vi "Call.vi"(7 "Actor in":refnum<class "Actor.lvclass">, 8 "Error in":errorcluster, 9 "Error":errorcluster, 10 "Actor":refnum<class "Actor.lvclass">) -> (0 "Error out":errorcluster, 5 "Actor out":refnum<class "Actor.lvclass">)   [LabVIEW 2025, in "jettl.lvlib" / "Stopped jettl Msg.lvlib"]
uses:
  Stopped jettl Msg.lvlib
  Stopped Msg/Stopped Msg/Stopped Msg.lvclass
  C:/git/jettl/src/jettl/jettl/Stopped jettl Msg/--Stopped Msg/Stopped Msg.lvclass
  C:/git/jettl/src/jettl/jettl/Msg/Msg.lvclass
  jettl.lvlib
  Stopped Msg Output/Stopped Msg Output/Stopped Msg Output.lvclass
  Actor/Actor.lvclass
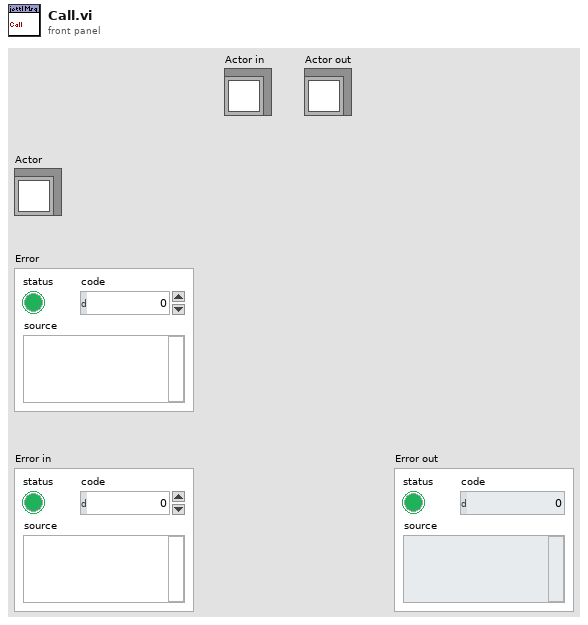
[diagram p1: front panel]
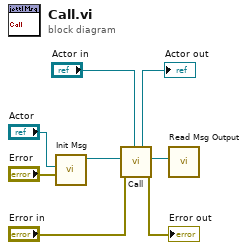
[diagram p0: block diagram]
diagram:
  n1 = call "Init Msg.vi"("Error"="Error", "Actor"="Actor") -> ("Stopped Msg out"=w6:refnum<class "Stopped Msg.lvclass">)  [unwired: 9 in]
  n2 = call "Call.vi"("Actor in"="Actor in", "Error in"="Error in", "Msg"=w6) -> ("Error out"=→"Error out":errorcluster, "Msg Output"=w2:refnum<class "Msg Output.lvclass">, "Actor out"=→"Actor out":refnum<class "Actor.lvclass">)  [unwired: 6 in]
  n3 = call "Read Msg Output.vi"("Msg Output"=w2) -> ()  [unwired: 11 in]
